vi "Autonomous Independent.vi"   [LabVIEW 2012]
doc: "This VI is called when autonomous begins, and will automatically be terminated when autonomous ends. You can carry out timed or sensor driven robot movement independently without needing to return to the caller."
uses:
  Robot Global Data.vi
types:
  T1 = typedef "WPI_MotorControlDeviceRef.ctl" = cluster{"DeviceStatus":errorcluster, "Type":enum16{"PWM", "CAN"}, "PWM":cluster{"Digital Module":T2, "PWM Channel":T3, "DeadBand":T4}, "CAN":cluster{"Device Number":u8, "Control Mode":T5, "Semaphore":T6, "Max Vout":dbl}, "Invert":bool, "TransformRef":T7, "InvTransformRef":T7}
  T2 = typedef "FPGA_TypedefDigitalModule.ctl" = enum16{"Digital Module 1", "Digital Module 2"}
  T3 = typedef "FPGA_DIOPWMChannel.ctl" = enum8{"PWM 1", "PWM 2", "PWM 3", "PWM 4", "PWM 5", "PWM 6", "PWM 7", "PWM 8", "PWM 9", "PWM 10", "Invalid"}
  T4 = typedef "WPI_PWMDeadband.ctl" = cluster{"Name":string, "maxPositivePwm":i32, "minPositivePwm":i32, "centerPwm":i32, "maxNegativePwm":i32, "minNegativePwm":i32, "angularRange":u16}
  T5 = typedef "WPI_CANJaguar_ControlMode.ctl" = enum8{"Percent VBus", "Current", "Speed", "Position", "Voltage"}
  T6 = typedef "Semaphore RefNum" = refnum<k1>
  T7 = typedef "WPI_PWMTransform_ConPane.ctl" = refnum<vi>
  T8 = typedef "WPI_GyroDevRef.ctl" = cluster{"DevStatus":errorcluster, "Analog Module":T9, "Analog Channel":T10, "Offset":dbl, "Gain (VoltsPerDegree/Second)":dbl}
  T9 = typedef "FPGA_TypedefAnalogModule.ctl" = enum16{"Analog Module 1", "Analog Module 2"}
  T10 = typedef "FPGA_AIChannel.ctl" = enum8{"AI 1", "AI 2", "AI 3", "AI 4", "AI 5", "AI 6", "AI 7", "AI 8", "Invalid"}
  T11 = typedef "WPI_EncoderDevRef.ctl" = cluster{"DevStatus":errorcluster, "EncoderIndex":T12, "CounterIndex":T13, "DistancePerCount":dbl, "Decoding Type":T14}
  T12 = typedef "FPGA_EncoderIdx.ctl" = enum8{"Enc 0", "Enc 1", "Enc 2", "Enc 3", "Invalid"}
  T13 = typedef "FPGA_CounterCtrSystemIndex.ctl" = enum8{"Ctr 0", "Ctr 1", "Ctr 2", "Ctr 3", "Ctr 4", "Ctr 5", "Ctr 6", "Ctr 7", "Invalid"}
  T14 = typedef "WPI_EncoderType.ctl" = enum16{"1x", "2x", "4x"}
  T15 = cluster{"Shifting":cluster{"Right Servo High":dbl, "Right Servo Low":dbl, "Left Servo High":dbl, "Left Servo Low":dbl}, "Breaking":cluster{"Coast Position":dbl, "Break Position":dbl}}
  T16 = cluster{"Right Servo High":dbl, "Right Servo Low":dbl, "Left Servo High":dbl, "Left Servo Low":dbl}
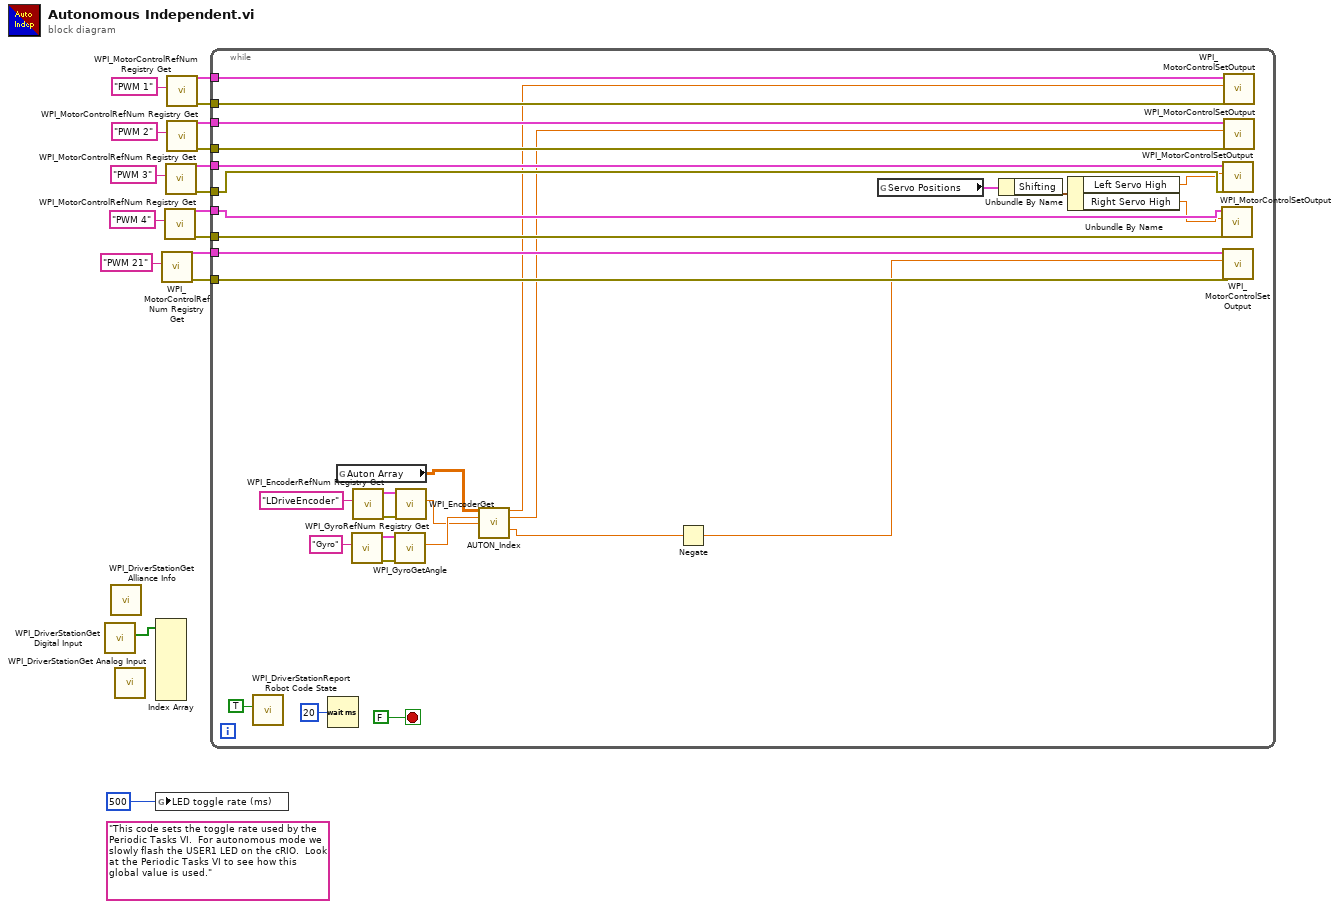
[diagram p0: block diagram]
diagram:
  (unwired) "This code sets the toggle rate used by the Periodic Tasks VI.  For autonomous mode we slowly flash the USER1 LED on the cRIO.  Look at the Periodic Tasks VI to see how this global value is used."
  n1 = call <vilib>:"WPI_DriverStationGet Digital Input.vi"() -> ("Driver Station Digital Input (1-8)"=w17:bool[])  [unwired: 11 out]
  n2 = call <vilib>:"WPI_DriverStationGet Alliance Info.vi"() -> ()  [unwired: 12 out]
  n3 = call <vilib>:"WPI_DriverStationGet Analog Input.vi"() -> ()  [unwired: 12 out]
  n4 = Index Array(array=w17) -> ()  [unwired: 8 in, 8 out]
  n5 = global write "Robot Global Data.vi" "LED toggle rate (ms)"(u32 500 ("LED ms toggle rate")) -> ()
  n6 = call <vilib>:"WPI_MotorControlRefNum Registry Get.vi"("refnum name"="PWM 21") -> ("error out"=w1:errorcluster, "MotorControlDevRef"=w2:T1)  [unwired: 9 in]
  n7 = call <vilib>:"WPI_MotorControlRefNum Registry Get.vi"("refnum name"="PWM 4") -> ("error out"=w6:errorcluster, "MotorControlDevRef"=w5:T1)  [unwired: 9 in]
  n8 = call <vilib>:"WPI_MotorControlRefNum Registry Get.vi"("refnum name"="PWM 3") -> ("error out"=w7:errorcluster, "MotorControlDevRef"=w8:T1)  [unwired: 9 in]
  n9 = call <vilib>:"WPI_MotorControlRefNum Registry Get.vi"("refnum name"="PWM 1") -> ("error out"=w13:errorcluster, "MotorControlDevRef"=w14:T1)  [unwired: 9 in]
  n10 = call <vilib>:"WPI_MotorControlRefNum Registry Get.vi"("refnum name"="PWM 2") -> ("error out"=w12:errorcluster, "MotorControlDevRef"=w11:T1)  [unwired: 9 in]
  n11 = while {
    tunnel: w14 -> [w44]
    tunnel: w13 -> [w43]
    tunnel: w11 -> [w41]
    tunnel: w12 -> [w42]
    tunnel: w8 -> [w40]
    tunnel: w7 -> [w39]
    tunnel: w5 -> [w37]
    tunnel: w6 -> [w38]
    tunnel: w2 -> [w27]
    tunnel: w1 -> [w26]
    stop <- FALSE stop-if-true
    n12 = call <vilib>:"WPI_DriverStationReport Robot Code State.vi"("Autonomous"=TRUE) -> ()  [unwired: 10 in, 1 out]
    n13 = Wait (ms)(milliseconds to wait=u32 20) -> ()  [unwired: 1 out]
    n14 = global read "Robot Global Data.vi" "Auton Array"() -> (w30:dbl[][])
    n15 = call <vilib>:"WPI_GyroRefNum Registry Get.vi"("refnum name"="Gyro") -> ("error out"=w34:errorcluster, "GyroDevRef"=w33:T8)  [unwired: 9 in]
    n16 = call <vilib>:"WPI_EncoderRefNum Registry Get.vi"("refnum name"="LDriveEncoder") -> ("error out"=w36:errorcluster, "EncoderDevRef"=w35:T11)  [unwired: 9 in]
    n17 = call <vilib>:"WPI_GyroGetAngle.vi"("error in (no error)"=w34, "GyroDevRef"=w33) -> ("Angle"=w29:dbl)  [unwired: 6 in, 3 out]
    n18 = call <vilib>:"WPI_EncoderGet.vi"("error in (no error)"=w36, "EncoderDevRef"=w35) -> ("Distance"=w28:dbl)  [unwired: 4 in, 5 out]
    n19 = call "AUTON_Index.vi"("Auton Array"=w30, "MeasuredHeading"=w29, "LeftEncoder"=w28) -> ("Left Drive"=w18:dbl, "Right Drive"=w19:dbl, "Shooter Elevation"=w25:dbl)  [unwired: 6 in, 4 out]
    n20 = Negate(x=w25) -> (-x=w24:dbl)
    n21 = global read "Robot Global Data.vi" "Servo Positions"() -> (w23:T15)
    n22 = Unbundle By Name(w23) -> ("Shifting"=w22:T16)
    n23 = Unbundle By Name(w22) -> ("Left Servo High"=w21:dbl, "Right Servo High"=w20:dbl)
    n24 = call <vilib>:"WPI_MotorControlSetOutput.vi"("error in (no error)"=w38, "Output"=w20, "MotorControlDevRef"=w37) -> ()  [unwired: 6 in, 3 out]
    n25 = call <vilib>:"WPI_MotorControlSetOutput.vi"("error in (no error)"=w39, "Output"=w21, "MotorControlDevRef"=w40) -> ()  [unwired: 6 in, 3 out]
    n26 = call <vilib>:"WPI_MotorControlSetOutput.vi"("error in (no error)"=w26, "Output"=w24, "MotorControlDevRef"=w27) -> ()  [unwired: 6 in, 3 out]
    n27 = call <vilib>:"WPI_MotorControlSetOutput.vi"("error in (no error)"=w43, "Output"=w18, "MotorControlDevRef"=w44) -> ()  [unwired: 6 in, 3 out]
    n28 = call <vilib>:"WPI_MotorControlSetOutput.vi"("error in (no error)"=w42, "Output"=w19, "MotorControlDevRef"=w41) -> ()  [unwired: 6 in, 3 out]
  }
